vi "To Pythonic - Dictionary.vi"(3 "Pythonic Values":string[](array[string]), 5 "Pythonic Keys":string[](array[string])) -> (1 "Dictionary":string)   [LabVIEW 2020, in "OPI.lvclass"]
doc: "Convert LabVIEW data into valid pythonic representation. \n\nThe input arrays of strings should be valid pythonic values created with previous calls to To Pythonic converter."
uses:
  OPI.lvclass
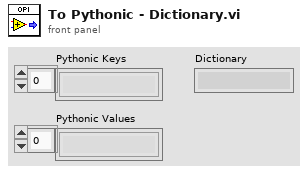
[diagram p1: front panel]
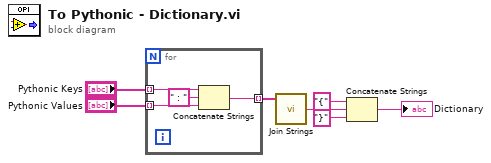
[diagram p0: block diagram]
diagram:
  n1 = for {
    tunnel: "Pythonic Keys" -> [w10] mode=indexing
    tunnel: "Pythonic Values" -> [w11] mode=indexing
    tunnel: [w8] -> w7 mode=indexing
    n2 = Concatenate Strings(w10, " : " ("string"), w11) -> (w8:string)
  }
  n3 = call <vilib>:"Join Strings.vi"("Strings In"=w7) -> ("String"=w6:string)  [unwired: 2 in]
  n4 = Concatenate Strings("{" ("string"), w6, "}" ("string")) -> (→"Dictionary":string)
